vi "Motion Chart Overlay test.vi"() -> ()   [LabVIEW 2017]
panel:
  out "Waveform Chart 4":dbl[][](graph)
  out "transposed array":dbl[][](array[numeric])
  out "Waveform Chart 3":dbl[](graph)
  out "Waveform Chart 2":dbl[][](graph)
  out "Waveform Graph":dbl[](graph)
  out "Waveform Chart":dbl(graph)
  in  "stop":bool
  in  "Motion Inputs":T1
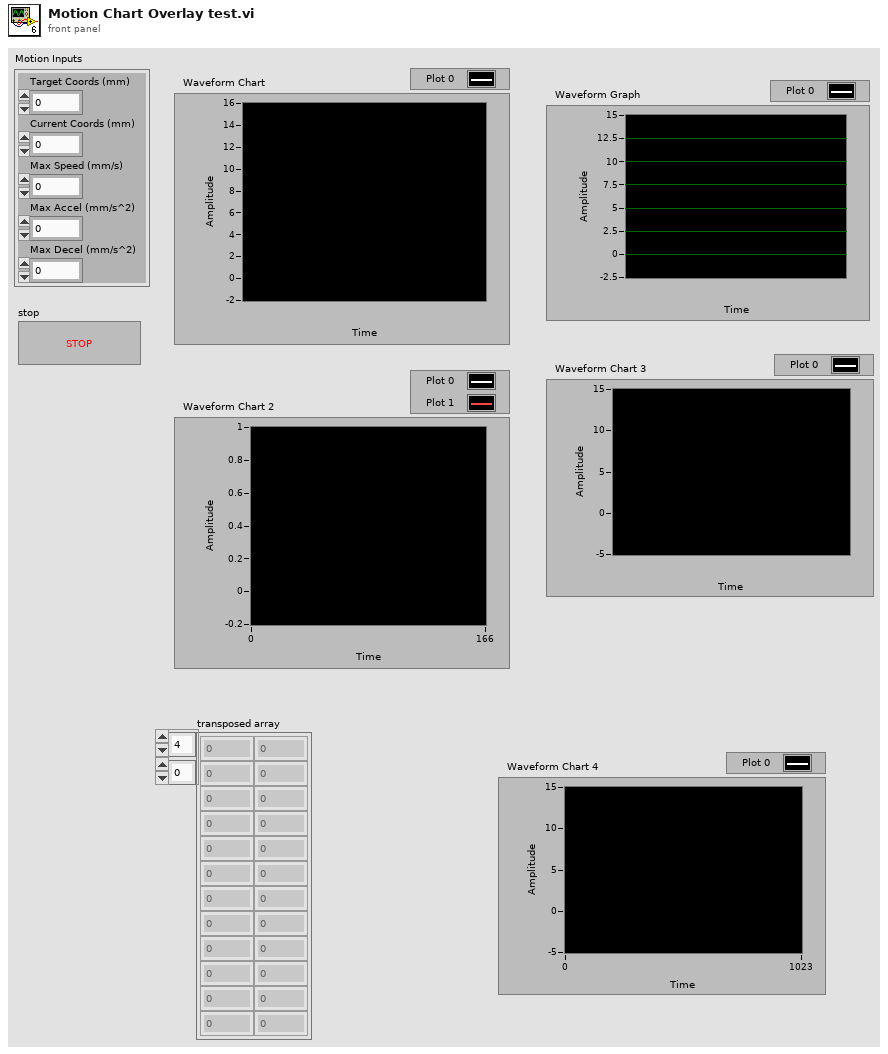
[diagram p1: front panel]
types:
  T1 = cluster{"Target Coords (mm)":dbl, "Current Coords (mm)":dbl, "Max Speed (mm/s)":dbl, "Max Accel (mm/s^2)":dbl, "Max Decel (mm/s^2)":dbl}
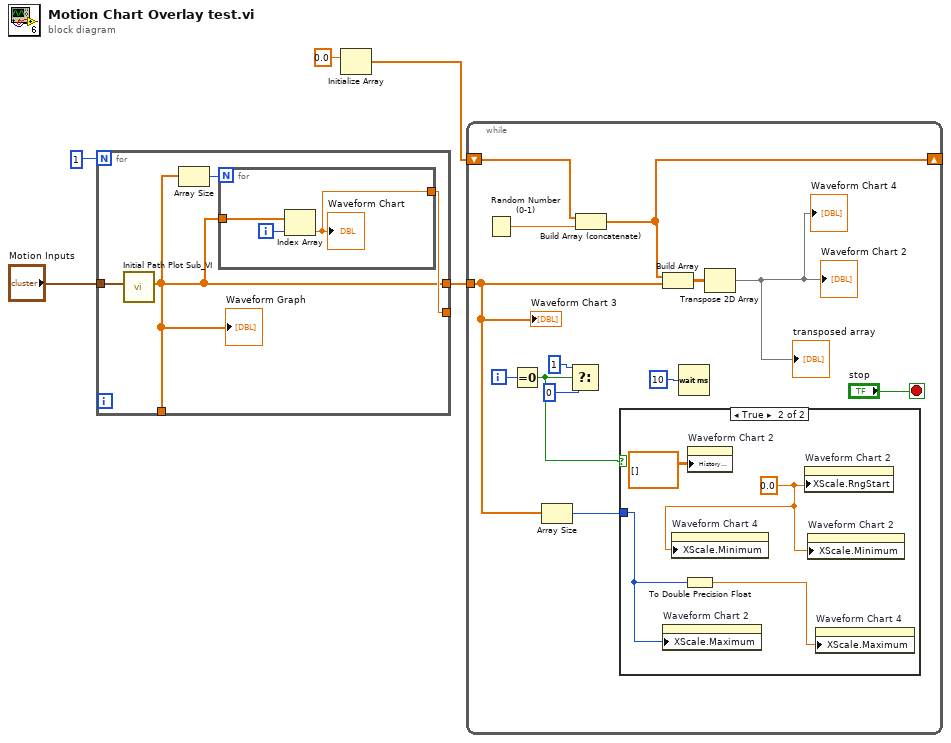
[diagram p0: block diagram]
diagram:
  n1 = for {
    N: 1 -> [_]
    tunnel: "Motion Inputs" -> [w9]
    tunnel: [w7] -> _
    tunnel: [w6] -> w1
    tunnel: [w6] -> _
    n2 = call "Initial Path Plot Sub_VI.vi"("Motion Inputs"=w9) -> ("Velocity Array"=w6:dbl[])  [unwired: 3 in, 7 out]
    "Waveform Graph" <- w6
    n3 = Array Size(array=w6) -> (size(s)=w8:i32)
    n4 = for {
      N: w8 -> [_]
      tunnel: w6 -> [w12]
      tunnel: [w10] -> w7
      i -> [w11]
      n5 = Index Array(array=w12, index=w11) -> (element=w10:dbl)
      "Waveform Chart" <- w10
    }
  }
  n6 = Initialize Array(0.0 ("element")) -> (w2:dbl[])  [unwired: 1 in]
  n7 = while {
    tunnel: w1 -> [w14]
    shift-right: [w19] -> _
    shift-left: w2 -> [w20]
    i -> [w17]
    stop <- "stop" stop-if-true
    n8 = Random Number (0-1)() -> (number: 0 to 1=w18:dbl)
    n9 = Equal To 0?(x=w17) -> (x = 0?=w16:bool)
    n10 = Array Size(array=w14) -> (size(s)=w13:i32)
    n11 = Select(t=1, s=w16, f=0) -> ()  [unwired: 1 out]
    n12 = Build Array (concatenate)(w20, w18) -> (w19:dbl[])
    n13 = case shown="True" w16 {
      tunnel: w13 -> [_ w27]
      frame False {
      }
      frame True {
        w26 = 0.0 ("X Scale.Range:Minimum")
        n14 = property on="Waveform Chart 2" class="WFChart (strict)"("XScale.Maximum"=w27) -> ()  [unwired: 2 in, 2 out]
        n15 = property on="Waveform Chart 4" class="WFChart (strict)"("XScale.Minimum"=w26) -> ()  [unwired: 2 in, 2 out]
        n16 = To Double Precision Float(number=w27) -> (double precision float=w28:dbl)
        n17 = property on="Waveform Chart 2" class="WFChart (strict)"("History Data"=dbl[][] []) -> ()  [unwired: 2 in, 2 out]
        n18 = property on="Waveform Chart 2" class="WFChart (strict)"("XScale.RngStart"=w26) -> ()  [unwired: 2 in, 2 out]
        n19 = property on="Waveform Chart 2" class="WFChart (strict)"("XScale.Minimum"=w26) -> ()  [unwired: 2 in, 2 out]
        n20 = property on="Waveform Chart 4" class="WFChart (strict)"("XScale.Maximum"=w28) -> ()  [unwired: 2 in, 2 out]
      }
    }
    n21 = Build Array(w19, w14) -> (w21:dbl[][])
    n22 = Wait (ms)(milliseconds to wait=u32 10) -> ()  [unwired: 1 out]
    n23 = Transpose 2D Array(2D array=w21) -> (transposed array=→"Waveform Chart 2" →"transposed array" →"Waveform Chart 4":dbl[][])
    "Waveform Chart 3" <- w14
  }
